vi "TOP LEVEL VI.vi"() -> ()   [LabVIEW 2013]
doc: "This Continuous Measurement sample project is based on the Queued Message Handler template.\n\nThe Event Handling Loop generates messages based on user interface actions.\n\nThe Message Handling Loop processes messages generated by the Event Handling Loop, or by other messages. There are also Acquisition and Logging message handling loop subVIs, and a chart updating loop."
uses:
  Typedefs/Objective selector control enum.ctl
  Typedefs/Laser control knob.ctl
  Typedefs/PMT control knob.ctl
  Typedefs/Frame Size.ctl
  Typedefs/AOL modes.ctl
  Peripherals Control/XYZ Stage/Typedefs/XYZ channel ring.ctl
  Typedefs/Plane Mode.ctl
  Typedefs/AVI implementation enum.ctl
  Typedefs/UI ctrl refs cluster.ctl
  User Interface/Typedefs/Next state queue data.ctl
  Typedefs/Start-Stop Enum.ctl
  Typedefs/Top level VI states.ctl
  Typedefs/Shutter Function Enum.ctl
  <vilib>/Utility/error.llb/DialogType.ctl
  Logging/Globals/gl_Binary timelapse files globals.vi
  Peripherals Control/Pockels/Globals/gl_Pockels control globals.vi
  Global Variables/General Globals.vi
  Global Variables/gl_UI Ctrl Refs.vi
panel:
  in  "Dummy button":bool
  in  "Speed Logging":bool
  in  "Time Lapse":bool
  in  "Live Imaging":bool
  in  "Axis":T1="All" caption="Axis to zero"
  in  "Return to Origin":bool
  out "Stage XYZ Position":cluster{"X":sgl, "Y":sgl, "Z":sgl} caption="Current Stage Position (µm)" {"Z" format="Z:%#_g"; "Y" format="Y:%#_g"; "X" format="X:%#_g"}
  out "Stop":bool=TRUE
  in  "Field of View":sgl(ring)=4.35 items=["175 um"=4.35, "250 um"=5.7, "350 um"=8.7]
  in  "AOL Mode":T2
  in  "Frame Size":T3=512 items=["100X100"=100, "128X128"=128, "200X200"=200, "256X256"=256, "512X512"=512, "1024x1024"=1024, "2048x2048"=2048]
  in  "Objective":T4="Olympus  20X"
  in  "Funct Acq button":bool
  in  "Motor Z Stack":bool
  in  "AOL Z Stack":bool
  in  "Exit button":bool
  in  "Imaging Param Tab":T5(tab)
  out "Power after objective (ind.)":dbl format="%#.0fmW"
  in  "Laser Power":T6=20 caption="LASER" max=1000 step=1 scale=0.0..100.0 scale format="%.0f%"
  out "Back aperture power (ind.)":dbl format="%#.0fmW"
  in  "AOL Z":sgl(slide) min=-178.5 max=177.65 step=0.01 scale=-178.5..177.65 scale format="%#_2f"
  in  "PMT 1":T7=550 max=1000 step=5 scale=0.0..1000.0
  in  "PMT 2":T7=550 max=1000 step=5 scale=0.0..1000.0
  in  "Averages":u16(knob) max=16 step=1 scale=0.0..16.0
  in  "Zoom":i8(slide)=1 min=1 max=24 step=1 scale=1.0..24.0
  in  "Dwell Time":dbl=0.10000000149011612 min=0.05 max=12.0 step=0.05000000074505806 format="%#.2fµs"
  out "Results Directory Overlay":string
  in  "Paths & Names":T8
  in  "Obtain Z Stop":bool
  in  "Obtain Z Start":bool
  in  "# Planes":u16=21 min=1 max=1000
  in  "Pockels@Z Stop":u16=5 caption="Laser % at Z Stop" max=100 format="%.0f%"
  in  "Pockels@Z Start":u16=5 caption="Laser % at Z Start" max=100 format="%.0f%"
  in  "Z Step":dbl=2.0 min=0.1 max=500.0 step=0.1 format="%#.1fµm"
  in  "Z Stop":dbl=-25.0 step=1.0 format="%#.0fµm"
  in  "Z Start":dbl=25.0 step=1.0 format="%#.0fµm"
  out "Center freq ind (nm)":dbl caption="Center frequency" min=800.0 max=1080.0 step=1.0 format="%#.2f MHz"
  in  "Enable f.acq post-processing":bool=TRUE
  in  "Video Record-Funct acq":bool
  in  "Video Record-Live Imaging":bool
  in  "Enable Video Recording":bool
  in  "Virtual Shutter":bool
  in  "Hard Shutter":bool
  in  "Plane Mode":T9 items=["XY Plane"]
  in  "Angle (degrees)":dbl caption="Angle" min=-180.0 max=180.0 format="%#_g°"
  in  "Y centre":dbl min=-1.0 max=1.0 step=0.1 format="%#.2f"
  in  "X centre":dbl min=-1.0 max=1.0 step=0.1 format="%#.2f"
  out "Laser wavelength ind (nm)":dbl caption="Laser wavelength" min=800.0 max=1080.0 step=1.0 format="%#.0f nm"
  in  "Live stim.trig.period":dbl=10.0 caption="Stimulus trigger period" min=0.001 max=50.0 step=1.0 format="%#.6f s"
  in  "Live stim.trig.enable":bool caption="Enable stimulus"
  in  "Funct. Acq. Pockels Modulation":bool caption="Pockels modulation"
  in  "AVI implementation":T10=enum."AVI2"
  in  "Snapshot":bool
  in  "Clear AOL GL":bool
  in  "Abort":bool caption="Stop"
  out "Last State (Ind.)":string
  in  "Switch user":bool
  out "Experiment folder path (ind.)":path caption="Generated experiment folder"
  out "Logging queue (ind)":i32 caption="Elements accumulating\nin the logging queue"
  out "AOL Z-stack Chirps Ready (ind)":bool
  out "Status ind":string
  # "Shutters"
  # "Post-Processing Options"
  # "Cameras Video Recording"
  # "Stimulus Trigger (Live protocols only)"
  # "Debugging Controls (Do not use)"
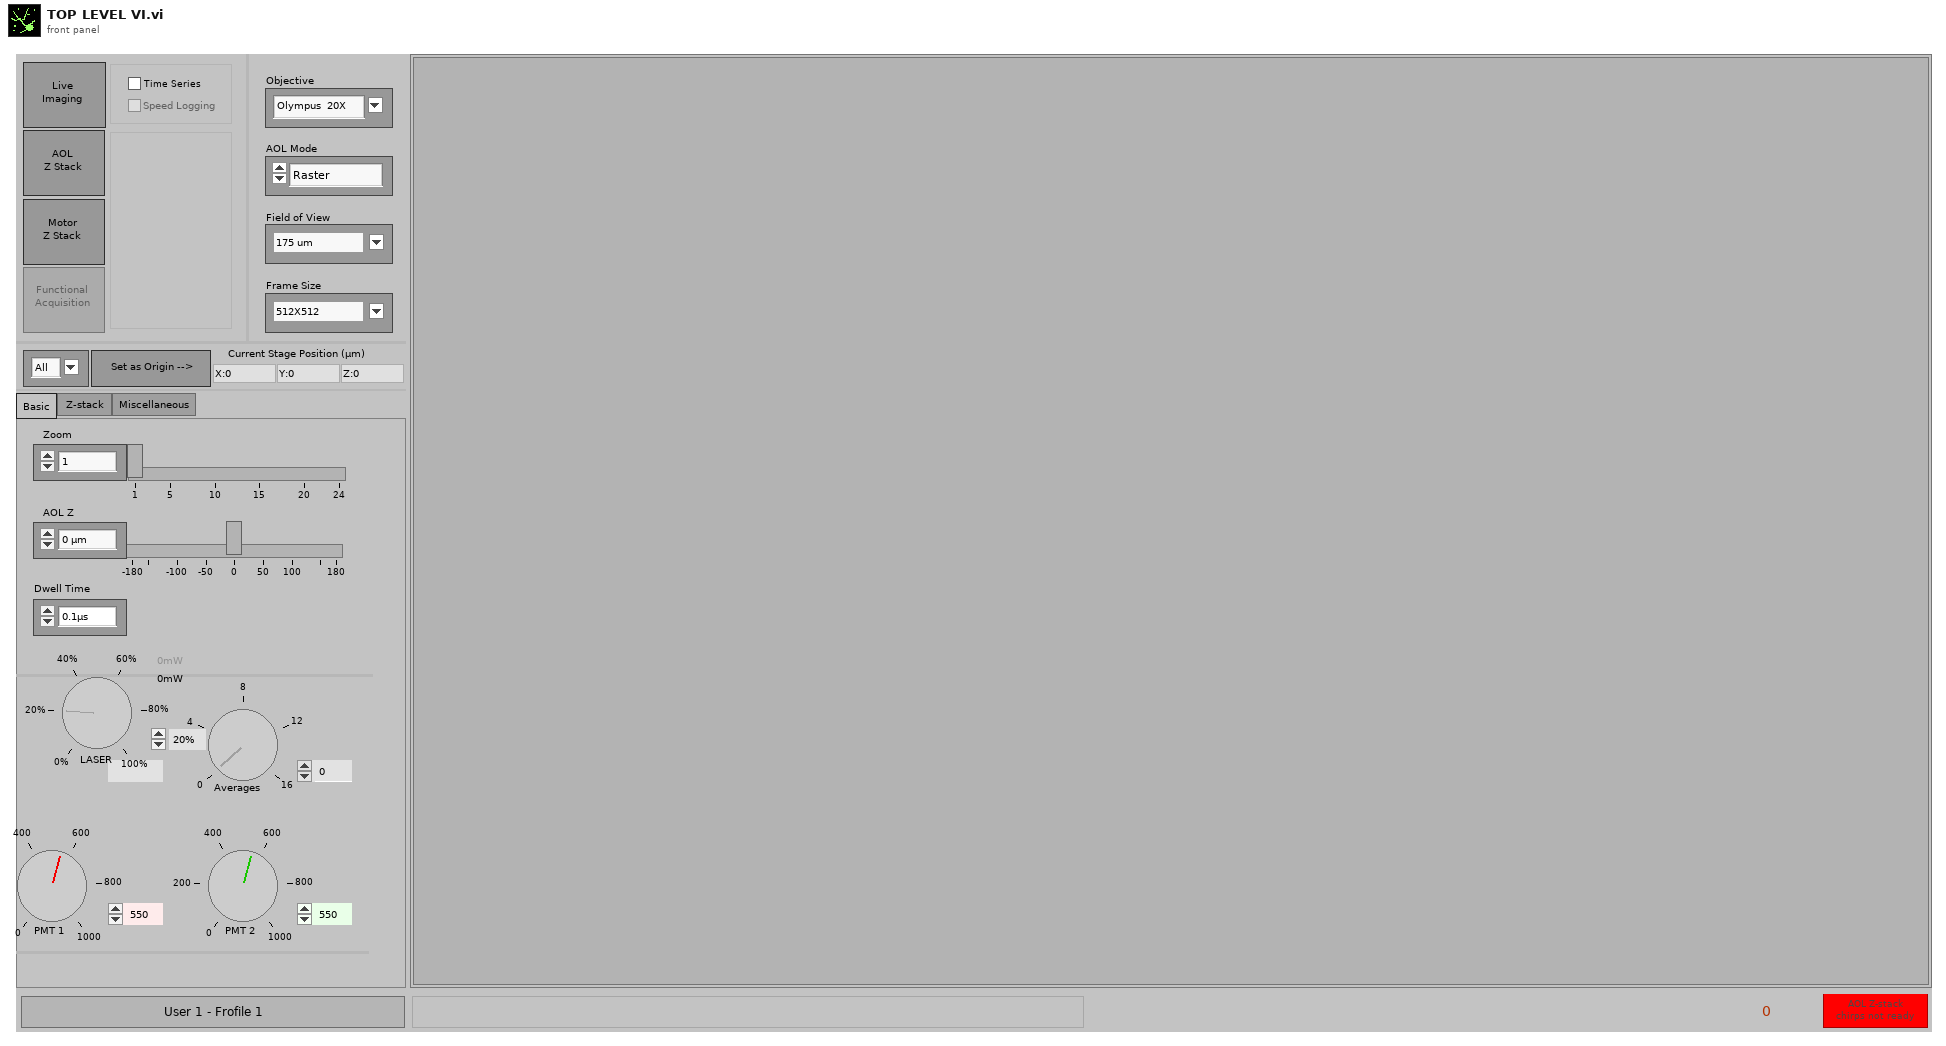
[diagram p1: front panel]
types:
  T1 = typedef "XYZ channel ring.ctl" = string
  T2 = typedef "AOL modes.ctl" = enum16{"Raster", "Structural", "Pointing", "Mini Scan", "Alignment"}
  T3 = typedef "Frame Size.ctl" = u16
  T4 = typedef "Objective selector control enum.ctl" = string
  T5 = enum32{"Basic", "Z-stack ", "Miscellaneous", "Development"}
  T6 = typedef "Laser control knob.ctl" = u16
  T7 = typedef "PMT control knob.ctl" = u16
  T8 = cluster{"Base Directory":path, "User folder?":bool, "Sub-Folder":string, "Experiment folder custom name":string}
  T9 = typedef "Plane Mode.ctl" = u16
  T10 = typedef "AVI implementation enum.ctl" = enum16{"AVI1", "AVI2"}
  T11 = typedef "UI ctrl refs cluster.ctl" = cluster{"Top level VI path":path, "Top level VI ref":refnum<vi>, "User menu ref":refnum<k9>, "Sub Panel control":refnum<vi>, "Imaging Param Tab":refnum<vi>, "Occurrence-Start drivers":refnum<k4>, "Occurrence-Speed logging initialised":refnum<k4>, "Occurrence-XYZ stage initialised":refnum<k4>, "Exit button":refnum<vi>, "Status ind":refnum<vi>, "Return to Origin":refnum<vi>, "Speed Logging":refnum<vi>, "Time Lapse":refnum<vi>, "Live Imaging":refnum<vi>, "AOL Z Stack":refnum<vi>, "Motor Z Stack":refnum<vi>, "Funct Acq button":refnum<vi>, "Hard Shutter":refnum<vi>, "Virtual Shutter":refnum<vi>, "Laser Power":refnum<vi>, "AOL Mode":refnum<vi>, "Frame Size":refnum<vi>, "Field of View":refnum<vi>, "Dwell Time":refnum<vi>, "Zoom":refnum<vi>, "AOL Z":refnum<vi>, "Objective":refnum<vi>, "Axis":refnum<vi>, "Paths & Names":refnum<vi>, "Experiment folder path (ind.)":refnum<vi>, "Last State (Ind.)":refnum<vi>, "Laser wavelength ind (nm)":refnum<vi>, "Averages":refnum<vi>, "Angle (degrees)":refnum<vi>, "X centre":refnum<vi>, "Y centre":refnum<vi>, "Plane Mode":refnum<vi>, "# Planes":refnum<vi>, "Z Start":refnum<vi>, "Z Stop":refnum<vi>, "Z Step":refnum<vi>, "PMT 1":refnum<vi>, "PMT 2":refnum<vi>, "Stage XYZ Position":refnum<vi>, "Pockels@Z Start":refnum<vi>, "Pockels@Z Stop":refnum<vi>, "Obtain Z Start":refnum<vi>, "Obtain Z Stop":refnum<vi>, "Live stim.trig.period":refnum<vi>, "Live stim.trig.enable":refnum<vi>, "Funct. Acq. Pockels Modulation":refnum<vi>, "Enable Video Recording":refnum<vi>, "Video Record-Live Imaging":refnum<vi>, "Video Record-Funct acq":refnum<vi>, "AOL Z-stack Chirps Ready (ind)":refnum<vi>, "Center freq ind (nm)":refnum<vi>, "Logging queue (ind)":refnum<vi>, "Back aperture power (ind.)":refnum<vi>, "Power after objective (ind.)":refnum<vi>, "Switch user":refnum<vi>}
  T12 = enum8{"Enabled", "Disabled", "Disabled and Grayed Out"}
  T13 = typedef "Next state queue data.ctl" = cluster{"Start/Stop":T14, "State":T15}
  T14 = typedef "Start-Stop Enum.ctl" = enum16{"START", "STOP"}
  T15 = typedef "Top level VI states.ctl" = enum16{"None", "Initialise UI", "<STACK PROTOCOL STATES>", "AOL Zstack-START", "AOL Zstack-STOP", "Motor Zstack-START", "Motor Zstack-STOP", "<ACQUISITION PROTOCOL STATES> ", "Functional Acquisition-START", "Functional Acquisition-STOP", "Single Plane Acquisition-START", "Single Plane Acquisition-STOP", "Volume Acquisition-START", "Volume Acquisition-STOP", "<LIVE IMAGING PROTOCOL STATES>", "Live Imaging-START", "Live Imaging-STOP", "Live Plane Imaging-START", "Live Plane Imaging-STOP", "Live Volume Imaging-START", "Live Volume Imaging-STOP", "EXIT"}
  T16 = enum16{"Write Red AVI", "Write Green AVI", "Write AVI mode"}
  T17 = typedef "Shutter Function Enum.ctl" = enum16{"Open Shutter", "Close Shutter"}
  T18 = enum16{"Software Init", "User menu", "Switch User button"}
  T19 = typedef "All Message Queues.ctl" = cluster{"UI queue":refnum<queue>, "Acq. queue":refnum<queue>, "Logging queue":refnum<queue>}
  T20 = typedef "DialogType.ctl" = u16
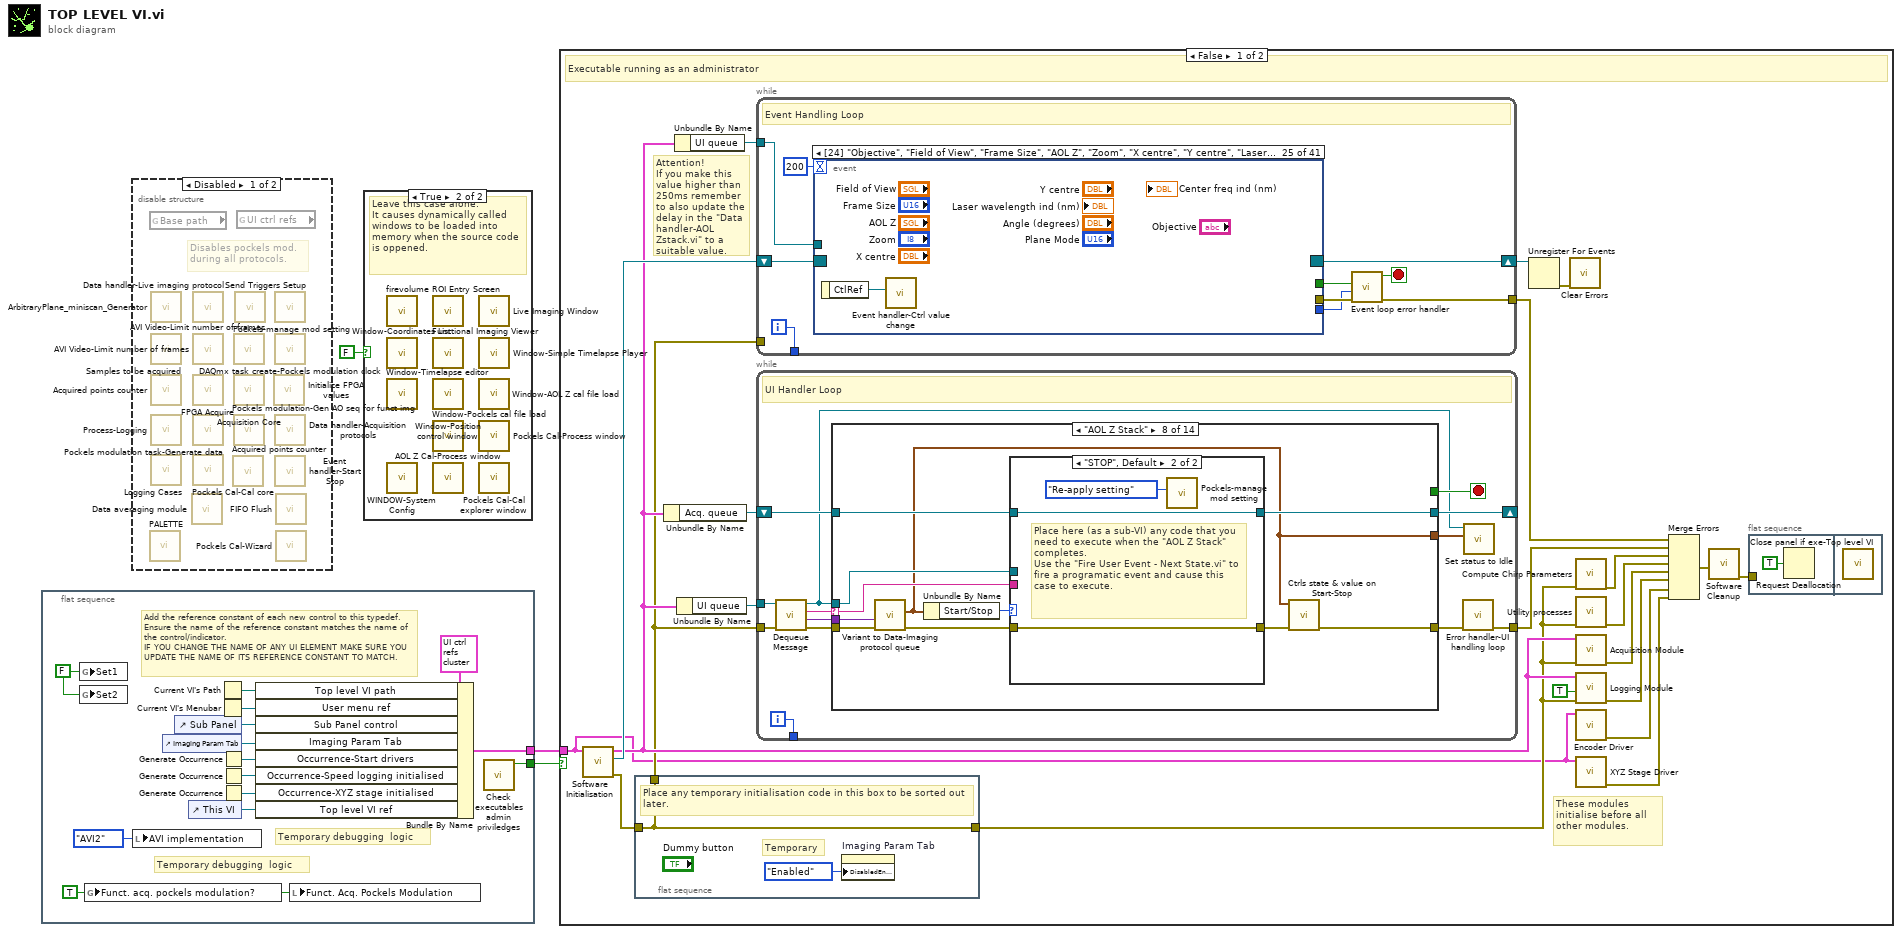
[diagram p0: block diagram]
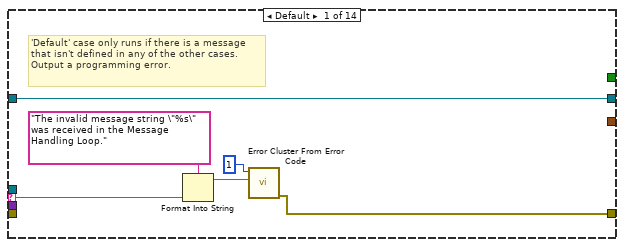
[diagram p2: hidden frame]
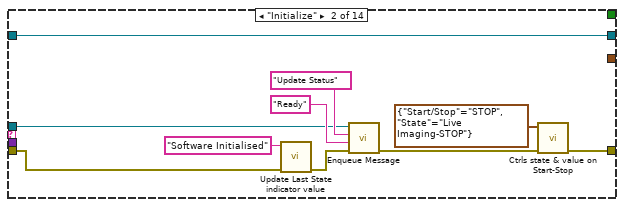
[diagram p3: hidden frame]
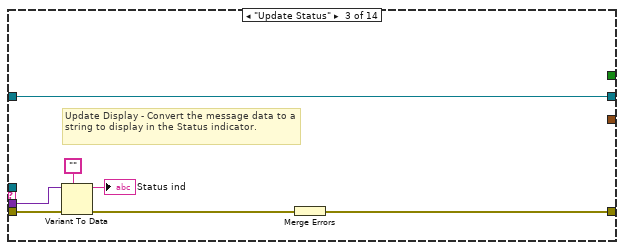
[diagram p4: hidden frame]
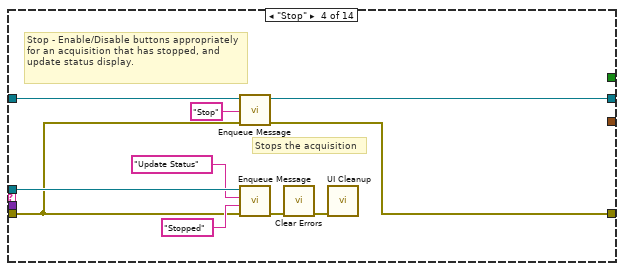
[diagram p5: hidden frame]
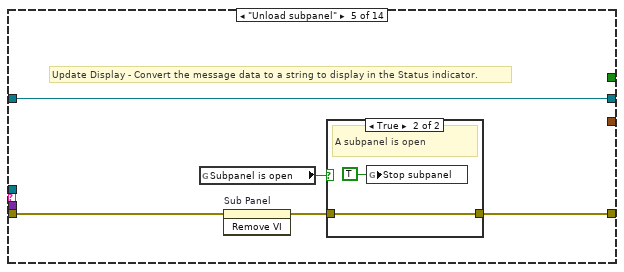
[diagram p6: hidden frame]
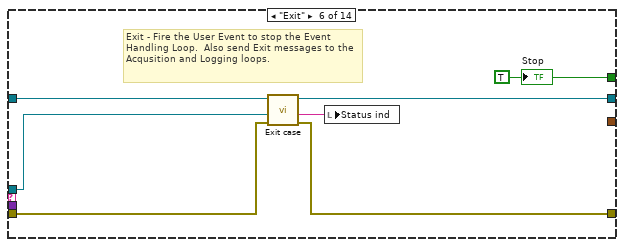
[diagram p8: hidden frame]
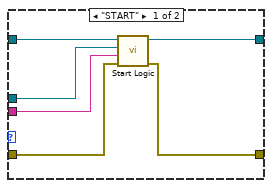
[diagram p10: hidden frame]
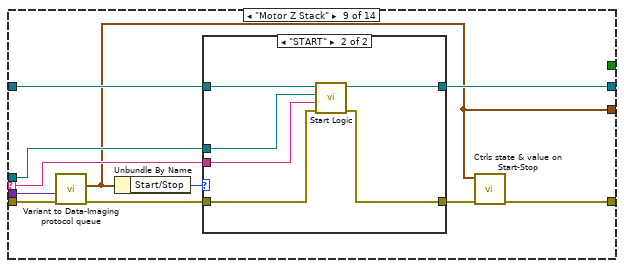
[diagram p11: hidden frame]
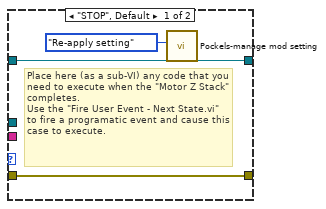
[diagram p12: hidden frame]
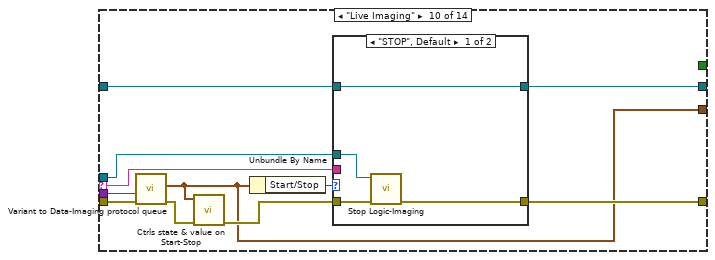
[diagram p13: hidden frame]
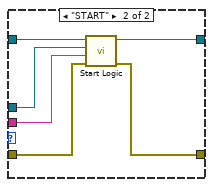
[diagram p14: hidden frame]
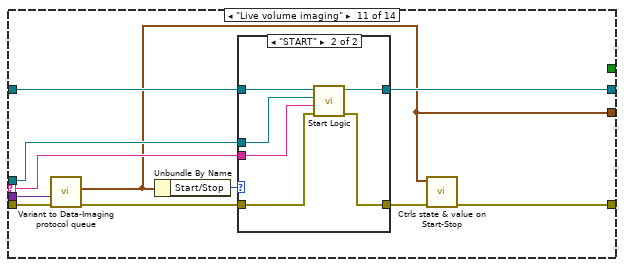
[diagram p15: hidden frame]
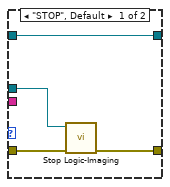
[diagram p16: hidden frame]
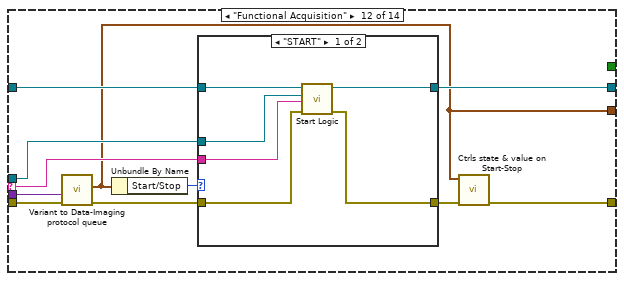
[diagram p17: hidden frame]
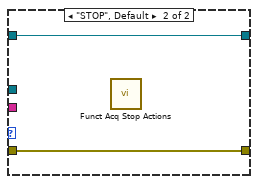
[diagram p18: hidden frame]
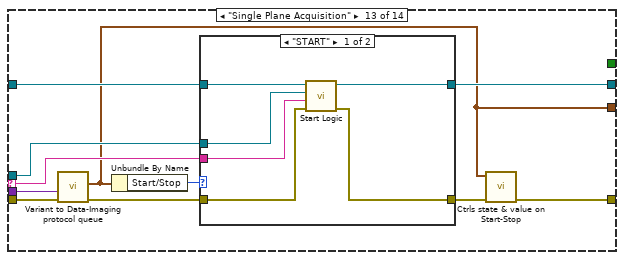
[diagram p19: hidden frame]
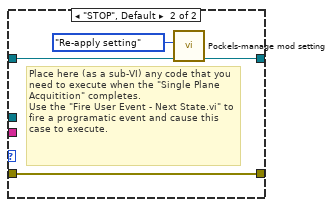
[diagram p20: hidden frame]
diagram:
  n1 = flat-sequence {
    tunnel: [w17] -> w2
    tunnel: [w4] -> w1
    frame #0 {
      w7 = TRUE ("Funct. acq. pockels modulation?")
      w9 = FALSE ("Set1")
      # "Temporary debugging  logic"
      # "Temporary debugging  logic"
      # "Add the reference constant of each new control to this typedef. Ensure the name of the reference constant matches the name of the control/indicator.\nIF YOU CHANGE THE NAME OF ANY UI ELEMENT MAKE SURE YOU UPDATE THE NAME OF ITS REFERENCE CONSTANT TO MATCH."
      n2 = global write "gl_Binary timelapse files globals.vi" "Set1"(w9) -> ()
      n3 = global write "gl_Binary timelapse files globals.vi" "Set2"(w9) -> ()
      n4 = global write "gl_Pockels control globals.vi" "Funct. acq. pockels modulation?"(w7) -> ()
      n5 = local write "AVI implementation"(AVI_implementation_enum."AVI2" ("AVI implementation")) -> ()
      n6 = control-ref of="Imaging Param Tab"() -> (w13:refnum<vi>)
      n7 = control-ref of="Sub Panel"() -> (w5:refnum<vi>)
      n8 = control-ref of="This VI"() -> (w10:refnum<vi>)
      n9 = Current VI's Path() -> (path=w15:path)
      n10 = Current VI's Menubar() -> (w16:refnum<k9>)
      n11 = Generate Occurrence() -> (w6:refnum<k4>)
      n12 = Generate Occurrence() -> (w11:refnum<k4>)
      n13 = Generate Occurrence() -> (w12:refnum<k4>)
      n14 = Bundle By Name(cluster=T11 {"Top level VI path"=path "", "Top level VI ref"=refnum, "User menu ref"=refnum, "Sub Panel control"=refnum, "Imaging Param Tab"=refnum, "Occurrence-Start drivers"=refnum, "Occurrence-Speed logging initialised"=refnum, "Occurrence-XYZ stage initialised"=refnum, "Exit button"=refnum, "Status ind"=refnum, "Return to Origin"=refnum, "Speed Logging"=refnum, "Time Lapse"=refnum, "Live Imaging"=refnum, "AOL Z Stack"=refnum, "Motor Z Stack"=refnum, "Funct Acq button"=refnum, "Hard Shutter"=refnum, "Virtual Shutter"=refnum, "Laser Power"=refnum, "AOL Mode"=refnum, "Frame Size"=refnum, "Field of View"=refnum, "Dwell Time"=refnum, "Zoom"=refnum, "AOL Z"=refnum, "Objective"=refnum, "Axis"=refnum, "Paths & Names"=refnum, "Experiment folder path (ind.)"=refnum, "Last State (Ind.)"=refnum, "Laser wavelength ind (nm)"=refnum, "Averages"=refnum, "Angle (degrees)"=refnum, "X centre"=refnum, "Y centre"=refnum, "Plane Mode"=refnum, "# Planes"=refnum, "Z Start"=refnum, "Z Stop"=refnum, "Z Step"=refnum, "PMT 1"=refnum, "PMT 2"=refnum, "Stage XYZ Position"=refnum, "Pockels@Z Start"=refnum, "Pockels@Z Stop"=refnum, "Obtain Z Start"=refnum, "Obtain Z Stop"=refnum, "Live stim.trig.period"=refnum, "Live stim.trig.enable"=refnum, "Funct. Acq. Pockels Modulation"=refnum, "Enable Video Recording"=refnum, "Video Record-Live Imaging"=refnum, "Video Record-Funct acq"=refnum, "AOL Z-stack Chirps Ready (ind)"=refnum, "Center freq ind (nm)"=refnum, "Logging queue (ind)"=refnum, "Back aperture power (ind.)"=refnum, "Power after objective (ind.)"=refnum, "Switch user"=refnum} ("output cluster"), "Top level VI path"=w15, "User menu ref"=w16, "Sub Panel control"=w5, "Imaging Param Tab"=w13, "Occurrence-Start drivers"=w6, "Occurrence-Speed logging initialised"=w11, "Occurrence-XYZ stage initialised"=w12, "Top level VI ref"=w10) -> (w17:T11)
      n15 = local write "Funct. Acq. Pockels Modulation"(w7) -> ()
      n16 = call "Check executables admin priviledges.vi"() -> ("Exe not run as an administrator"=w4:bool)  [unwired: 10 in, 1 out]
    }
  }
  n17 = disable-structure shown="Disabled" {
    frame Disabled {
      # "Disables pockels mod.\nduring all protocols."
      n18 = global read "General Globals.vi" "Base path"() -> ()  [unwired: 1 out]
      n19 = call "PALETTE.vi"() -> ()  [unwired: 12 in]
      n20 = call "ArbitraryPlane_miniscan_Generator.vi"() -> ()  [unwired: 7 in, 5 out]
      n21 = call "Samples to be acquired.vi"() -> ()  [unwired: 10 in, 2 out]
      n22 = call "Acquired points counter.vi"() -> ()  [unwired: 12 in, 4 out]
      n23 = call "Process-Logging.vi"() -> ()  [unwired: 11 in, 1 out]
      n24 = call "Logging Cases.vi"() -> ()  [unwired: 14 in, 2 out]
      n25 = call "Data averaging module.vi"() -> ()  [unwired: 8 in, 4 out]
      n26 = call "Data handler-Live imaging protocol.vi"() -> ()  [unwired: 15 in, 1 out]
      n27 = call "AVI Video-Limit number of frames.vi"() -> ()  [unwired: 1 in, 1 out]
      n28 = call "FPGA Acquire.vi"() -> ()  [unwired: 11 in, 5 out]
      n29 = call "Pockels modulation task-Generate data.vi"() -> ()  [unwired: 7 in, 5 out]
      n30 = call "Pockels Cal-Cal core.vi"() -> ()  [unwired: 9 in, 3 out]
      n31 = call "Acquired points counter.vi"() -> ()  [unwired: 12 in, 4 out]
      n32 = call "AVI Video-Limit number of frames.vi"() -> ()  [unwired: 1 in, 1 out]
      n33 = call "Acquisition Core.vi"() -> ()  [unwired: 10 in, 2 out]
      n34 = call "Pockels modulation-Gen AO seq for funct img.vi"() -> ()  [unwired: 8 in, 4 out]
      n35 = call "Pockels-manage mod setting.vi"() -> ()  [unwired: 11 in, 1 out]
      n36 = global read "gl_UI Ctrl Refs.vi" "UI ctrl refs"() -> ()  [unwired: 1 out]
      n37 = call "Initialize FPGA values.vi"() -> ()  [unwired: 10 in, 2 out]
      n38 = call "Send Triggers Setup.vi"() -> ()  [unwired: 10 in, 2 out]
      n39 = call "DAQmx task create-Pockels modulation clock.vi"() -> ()  [unwired: 10 in, 2 out]
      n40 = call "Data handler-Acquisition protocols.vi"() -> ()  [unwired: 14 in, 2 out]
      n41 = call "Event handler-Start Stop.vi"() -> ()  [unwired: 10 in, 2 out]
      n42 = call "FIFO Flush.vi"() -> ()  [unwired: 9 in, 3 out]
      n43 = call "Pockels Cal-Wizard.vi"() -> ()  [unwired: 12 in]
    }
    frame Enabled {
    }
  }
  n44 = case shown="True" FALSE {
    frame False {
    }
    frame True {
      # "Leave this case alone.\nIt causes dynamically called windows to be loaded into memory when the source code is oppened."
      n45 = call "firevolume.vi"() -> ()  [unwired: 12 in]
      n46 = call "Window-Coordinates List.vi"() -> ()  [unwired: 12 in]
      n47 = call "Window-Timelapse editor.vi"() -> ()  [unwired: 12 in]
      n48 = call "WINDOW-System Config.vi"() -> ()  [unwired: 12 in]
      n49 = call "ROI Entry Screen.vi"() -> ()  [unwired: 12 in]
      n50 = call "Functional Imaging Viewer.vi"() -> ()  [unwired: 12 in]
      n51 = call "Window-Position control window.vi"() -> ()  [unwired: 12 in]
      n52 = call "Window-Pockels cal file load.vi"() -> ()  [unwired: 12 in]
      n53 = call "AOL Z Cal-Process window.vi"() -> ()  [unwired: 9 in, 3 out]
      n54 = call "Live Imaging Window.vi"() -> ()  [unwired: 12 in]
      n55 = call "Window-Simple Timelapse Player.vi"() -> ()  [unwired: 12 in]
      n56 = call "Window-AOL Z cal file load.vi"() -> ()  [unwired: 12 in]
      n57 = call "Pockels Cal-Process window.vi"() -> ()  [unwired: 10 in, 2 out]
      n58 = call "Pockels Cal-Cal explorer window.vi"() -> ()  [unwired: 12 in]
    }
  }
  n59 = case shown="False" w1 {
    tunnel: w2 -> [w18 w319]
    frame False {
      # "These modules initialise before all other modules."
      # "Attention!\nIf you make this value higher than 250ms remember to also update the delay in the \"Data handler-AOL Zstack.vi\" to a suitable value."
      # "Executable running as an administrator"
      n60 = call "Software Initialisation.vi"("UI elements cluster"=w18) -> ("Error Out"=w37:errorcluster, "Event Registration Refnum"=w39:refnum<event-registration>, "Message Queues out"=w38:T19)  [unwired: 8 in]
      n61 = flat-sequence {
        tunnel: w37 -> [w41]
        tunnel: [w41] -> w21
        tunnel: [w41] -> w20
        frame #0 {
          # "Temporary"
          # "Place any temporary initialisation code in this box to be sorted out later."
          n62 = property on="Imaging Param Tab" class="TabCtl (strict)"("DisabledEnum"=T12."Enabled" ("Disabled")) -> ()  [unwired: 2 in, 2 out]
        }
      }
      n63 = Unbundle By Name(w38) -> ("Acq. queue"=w33:refnum<queue>)
      n64 = Unbundle By Name(w38) -> ("UI queue"=w35:refnum<queue>)
      n65 = Unbundle By Name(w38) -> ("UI queue"=w34:refnum<queue>)
      n66 = while {
        tunnel: w35 -> [w253]
        tunnel: [w251] -> w26
        shift-right: [w252] -> w36
        shift-left: w39 -> [w254]
        tunnel: [w248] -> _
        tunnel: w21 -> [_]
        i -> [w248]
        stop <- w256 stop-if-true
        # "Event Handling Loop"
        n67 = event shown="[24] \"Objective\", \"Field of View\", \"Frame Size\", \"AOL Z\", \"Zoom\", \"X centre\", \"Y centre\", \"Laser wavelength ind (nm)\", \"Angle (degrees)\", \"Plane Mode\": Value Change" {
          selector: w254 -> [_ _ _ _ _ _ _ _ _ _ _ _ _ _ _ _ _ _ _ _ _ _ _ _ _ _ _ _ _ _ _ _ _ _ _ _ _ _ _ _ _]
          dyn-events: [_ _ _ _ _ _ _ _ _ _ _ _ _ _ _ _ _ _ _ _ _ _ _ _ _ _ _ _ _ _ _ _ _ _ _ _ _ _ _ _ _] -> w252
          timeout: 200 -> [_ _ _ _ _ _ _ _ _ _ _ _ _ _ _ _ _ _ _ _ _ _ _ _ _ _ _ _ _ _ _ _ _ _ _ _ _ _ _ _ _]
          tunnel: [_ _ _ _ _ _ _ _ _ _ _ _ _ _ _ _ _ _ _ _ _ _ _ _ _ _ _ _ _ _ _ _ _ _ _ _ _ _ TRUE ("Discard?") _ _] -> w249
          tunnel: w253 -> [_ w258 _ _ w263 _ _ _ _ _ _ _ _ _ _ _ _ _ _ _ _ _ _ _ _ _ _ _ _ _ _ _ _ _ _ _ _ w311 _ w314 w317]
          tunnel: [_ w257 _ _ w262 _ _ _ w268 w273 w275 w277 _ _ w281 _ _ _ _ _ _ _ _ _ _ _ _ _ _ _ _ _ _ _ _ _ _ w310 _ w315 w318] -> w255
          tunnel: [_ _ _ _ w261 _ _ _ _ _ _ _ _ _ _ _ _ _ _ _ _ _ _ _ _ _ _ _ _ _ _ _ _ _ _ _ _ _ _ _ _] -> w247
          event Timeout {
            n68 = event-data() -> ()  [unwired: 1 in, 1 out]
          }
          event Menu Selection (User); "Experiment folder path (ind.)", "Results Directory Overlay": Shortcut Menu Selection (User) {
            n69 = event-data() -> ("ItemTag"=w259:string)  [unwired: 1 in]
            n70 = call "User menu handler.vi"("UI queue"=w258, "User Menu ItemTag"=w259) -> ("error out"=w257:errorcluster)  [unwired: 9 in]
          }
          event "Live stim.trig.period", "Return to Origin", "Laser wavelength ind (nm)": Shortcut Menu Selection (User) {
            n71 = event-data() -> ("ItemTag"=w260:string)  [unwired: 1 in]
            n72 = call "Top level UI-Shortcut menus handler.vi"("ItemTag"=w260) -> ()  [unwired: 11 in]
          }
          event Menu Activation? {
            n73 = event-data() -> ()  [unwired: 1 in, 5 out]
            n74 = call "menu-Cal group disabled state.vi"() -> ()  [unwired: 10 in, 2 out]
            n75 = event-data() -> ()  [unwired: 2 in, 1 out]
          }
          event User Event {
            # "Causes the \"UI Handler Loop\" to execute one of its cases. There are redundant cases as a provision.\nThis functionality is fully scalable and flexible allowing to programatically fire events from anywhere within the software, as well as when the user presses a button.\nThis event case also executes in response to a programmatic event which occurs when the user closes the ROI Entry Screen, and executes the required case, depending on which button the user pressed to exit the ROI Entry Screen."
            n76 = event-data() -> ("Next State"=w261:T15)  [unwired: 1 in]
            n77 = call "Event handler-Start Stop.vi"("Next State"=w261, "UI queue"=w263) -> ("error out"=w262:errorcluster)  [unwired: 8 in, 1 out]
          }
          event "Experiment folder path (ind.)": Shortcut Menu Activation? {
            n78 = event-data() -> ("CtlRef"=w266:refnum<vi>)  [unwired: 1 in]
            n79 = property class="Path"(reference=w266) -> ("Value"=w265:path)  [unwired: 1 in, 2 out]
            n80 = Empty String/Path?(string/path=w265) -> (empty?=w264:bool)
            n81 = event-data("Discard?"=w264) -> ()  [unwired: 1 in, 1 out]
          }
          event "Live stim.trig.enable", "Live stim.trig.period": Value Change {
            n82 = event-data() -> ()  [unwired: 1 in, 1 out]
            n83 = call "Stimulus trigger period event handler.vi"() -> ()  [unwired: 12 in]
          }
          event "Enable f.acq post-processing": Value Change {
            n84 = event-data() -> ("NewVal"=w267:bool)  [unwired: 1 in]
            n85 = global write "General Globals.vi" "Funct.acq post-proc enabled"(w267) -> ()
          }
          event "Live Imaging": Value Change {
            # "Sends the \" <Next state>:User Event \" case of this event structure to its specified sub-case."
            n86 = event-data() -> ("NewVal"=w272:bool)  [unwired: 1 in]
            n87 = Select(t=Top_level_VI_states."Live Imaging-START" ("event data / imaging mode"), s=w272, f=Top_level_VI_states."Live Imaging-STOP" ("event data / imaging mode")) -> (s? t:f=w270:T15)
            n88 = call "Fire User Event - Next State.vi"("\"UI Handler loop\" case to execute"=w270) -> ("Error Out"=w268:errorcluster)  [unwired: 10 in]
          }
          event "AOL Z Stack": Value Change {
            n89 = event-data() -> ("NewVal"=w274:bool)  [unwired: 1 in]
            n90 = call "Event handler-AOL Z button.vi"("AOL Z button's value"=w274) -> ("error out"=w273:errorcluster)  [unwired: 10 in]
          }
          event "Motor Z Stack": Value Change {
            n91 = event-data() -> ("NewVal"=w276:bool)  [unwired: 1 in]
            n92 = call "Event handler-Motor Z button.vi"("Motor Z button's value"=w276) -> ("error out"=w275:errorcluster)  [unwired: 10 in]
          }
          event "Funct Acq button": Value Change {
            n93 = event-data() -> ("NewVal"=w278:bool)  [unwired: 1 in]
            n94 = call "Event handler-Funct Acq button.vi"("Funct.Acq button's value"=w278) -> ("error out"=w277:errorcluster)  [unwired: 10 in]
          }
          event "Paths & Names.Base Directory": Value Change {
            n95 = event-data() -> ("OldVal"=w279:path)  [unwired: 1 in]
            n96 = call "Event handler-Dir change.vi"("Old Base Path"=w279) -> ()  [unwired: 11 in]
          }
          event "Paths & Names.User folder?": Value Change {
            n97 = event-data() -> ("NewVal"=w280:bool)  [unwired: 1 in]
            n98 = global write "General Globals.vi" "Generate user folder?"(w280) -> ()
          }
          event "Time Lapse": Value Change {
            n99 = event-data() -> ()  [unwired: 1 in, 1 out]
            n100 = call "Event handler-Timelapse.vi"() -> ("error out"=w281:errorcluster)  [unwired: 11 in]
          }
          event "Enable Video Recording": Value Change {
            n101 = event-data() -> ("NewVal"=w282:bool)  [unwired: 1 in]
            n102 = call "Event handler-VidRec enable.vi"("Enable Video Recording.NewVal"=w282) -> ()  [unwired: 11 in]
          }
          event "Video Record-Live Imaging": Value Change {
            n103 = event-data() -> ("NewVal"=w283:bool)  [unwired: 1 in]
            n104 = call "Event handler-VidRec enable in timelapse.vi"("Video Record-Live Imaging.NewVal"=w283) -> ()  [unwired: 11 in]
          }
          event "Video Record-Funct acq": Value Change {
            n105 = event-data() -> ("NewVal"=w284:bool)  [unwired: 1 in]
            n106 = call "Event handler-VidRec enable in funct.vi"("Video Record-Funct acq.NewVal"=w284) -> ()  [unwired: 11 in]
          }
          event Value Change {
            n107 = event-data() -> ("NewVal"=w285:T10)  [unwired: 1 in]
            n108 = call "fgv_AVI_Globals.vi"("AVI mode"=w285, "Function"=enum16{"Intialize", "Write", "Read", "Clear"}."Write", "\"Write\" sub function"=T16."Write AVI mode" ("\"Write\" sub function")) -> ()  [unwired: 9 in, 4 out]
          }
          event "Snapshot": Value Change {
            # "Warning! Redundant case. Eliminate if no longer needed."
            n109 = event-data() -> ()  [unwired: 1 in, 1 out]
            n110 = disable-structure shown="Disabled" {
              frame Disabled {
                # "Right graph data"
                # "Left graph data"
                # "As soon as this button is pressed this code grabs both the left and right graph data (each being a 2D array of points) and saves it to the file specified by the user in a pop up file-dialogue window."
                n111 = call "Intensity Graphs to Excel.vi"() -> ()  [unwired: 12 in]
              }
              frame Enabled {
              }
            }
          }
          event "Obtain Z Start", "Obtain Z Stop", "Z Step", "Z Start", "Z Stop": Value Change {
            n112 = event-data() -> ()  [unwired: 1 in, 1 out]
            n113 = call "Event handler-Z Setup.vi"("Obtain Z Stop"="Obtain Z Stop", "Obtain Z Start"="Obtain Z Start") -> ()  [unwired: 9 in, 1 out]
          }
          event "Pockels@Z Start", "Pockels@Z Stop": Value Change {
            n114 = event-data() -> ()  [unwired: 1 in, 1 out]
            n115 = call "Event handler-Z Setup pockels entry.vi"() -> ()  [unwired: 11 in, 1 out]
          }
          event "# Planes": Value Change {
            n116 = event-data() -> ()  [unwired: 1 in, 1 out]
            n117 = call "Event handler-Number of planes change.vi"() -> ()  [unwired: 11 in, 1 out]
          }
          event "Averages": Value Change {
            n118 = event-data() -> ("NewVal"=w290:u16)  [unwired: 1 in]
            n119 = call "Event handler-Averages ValChange.vi"("Averages.NewVal"=w290) -> ()  [unwired: 11 in]
          }
          event "Field of View", "AOL Z", "Zoom", "X centre", "Y centre", "Laser wavelength ind (nm)", "Angle (degrees)": Value Change {
            n120 = event-data() -> ("CtlRef"=w291:refnum<vi>)  [unwired: 1 in]
            n121 = call "Event handler-Ctrl value change.vi"("Control in"=w291) -> ()  [unwired: 11 in]
          }
          event "Dwell Time": Value Change {
            n122 = event-data() -> ()  [unwired: 1 in, 1 out]
            n123 = call "AOL Globals Dwell Time updater.vi"() -> ()  [unwired: 11 in, 1 out]
          }
          event Value Change {
            n124 = event-data() -> ()  [unwired: 1 in, 1 out]
            n125 = call "AOL Globals mode updater.vi"() -> ("error out"=w292:errorcluster)  [unwired: 11 in]
            n126 = call "AOL Globals Dwell Time updater.vi"("error in"=w292) -> ()  [unwired: 10 in, 1 out]
          }
          event "Return to Origin": Value Change {
            n127 = event-data() -> ()  [unwired: 1 in, 1 out]
            n128 = call "Event handler-Set coordinates to zero.vi"() -> ()  [unwired: 12 in]
          }
          event "Hard Shutter": Value Change {
            n129 = event-data() -> ()  [unwired: 1 in, 1 out]
            n130 = Select(t=Shutter_Function_Enum."Open Shutter" ("Shutter Function"), s="Hard Shutter", f=Shutter_Function_Enum."Close Shutter" ("Shutter Function")) -> (s? t:f=w294:T17)
            n131 = call "Set Hard Shutter.vi"("Shutter Function"=w294) -> ("Error Out"=w293:errorcluster)  [unwired: 10 in]
            n132 = case shown="Error" w293 {
              selector: w293 -> [_ w299]
              frame No Error {
              }
              frame Error {
                w300 = T20 0 items=["no dialog", "OK message", "continue or stop message", "OK message + warnings", "continue/stop + warnings"] ("type of dialog (OK msg:1)")
                n133 = call <vilib>:"Simple Error Handler.vi"("type of dialog (OK msg:1)"=w300, "error in (no error)"=w299) -> ("error out"=w298:errorcluster)  [unwired: 3 in, 4 out]
                n134 = call "Window-Error message.vi"("error in (no error)"=w298, "Message"="Hard shutter error") -> ()  [unwired: 9 in, 1 out]
              }
            }
          }
          event Value Change {
            n135 = event-data() -> ("NewVal"=w302:T6)  [unwired: 1 in]
            n136 = call "Event handler-Laser power value change.vi"("Laser Power knob.NewVal"=w302) -> ()  [unwired: 11 in]
          }
          event Mouse Up; Mouse Leave {
            n137 = event-data() -> ()  [unwired: 1 in, 1 out]
            n138 = local read "Laser Power"() -> (w304:T6)
            n139 = To Unsigned Byte Integer(number=w304) -> (unsigned 8bit integer=w303:u8)
            n140 = call "Set laser power.vi"("Laser power %"=w303) -> ()  [unwired: 10 in, 1 out]
          }
          event "Funct. Acq. Pockels Modulation": Value Change {
            n141 = event-data() -> ()  [unwired: 1 in, 1 out]
            n142 = global write "gl_Pockels control globals.vi" "Funct. acq. pockels modulation?"("Funct. Acq. Pockels Modulation") -> ()
          }
          event "Virtual Shutter": Value Change {
            n143 = event-data() -> ("NewVal"=w306:bool)  [unwired: 1 in]
            n144 = call "Event handler-Virtual shutter change.vi"("Virtual shutter button value"=w306) -> ()  [unwired: 11 in]
          }
          event Value Change {
            n145 = event-data() -> ()  [unwired: 1 in, 1 out]
            n146 = call "Event handler-PMT value change.vi"() -> ()  [unwired: 12 in]
          }
          event "Speed Logging": Value Change {
            n147 = event-data() -> ("NewVal"=w307:bool)  [unwired: 1 in]
            n148 = global write "General Globals.vi" "Speed logging enabled"(w307) -> ()
          }
          event "Clear AOL GL": Value Change {
            # "This functionality is only needed during development and it will be eventually eliminated."
            n149 = event-data() -> ()  [unwired: 1 in, 1 out]
            n150 = call "fgv_AOL_Globals.vi"("Function"=enum16{"Intialize", "Write", "Read", "Clear"}."Clear") -> ()  [unwired: 9 in, 2 out]
          }
          event "Switch user": Value Change {
            n151 = event-data() -> ()  [unwired: 1 in, 2 out]
            n152 = call "UsrProfiles-User login.vi"("Access source (Soft init)"=T18."Switch User button") -> ()  [unwired: 10 in, 1 out]
          }
          event "Abort": Value Change {
            n153 = event-data() -> ()  [unwired: 1 in, 1 out]
            n154 = call "Enqueue Message.vi"("Message"="Stop", "Queue"=w311) -> ("error out"=w310:errorcluster)  [unwired: 8 in, 1 out]
          }
          event User Event {
            # "Do not add any code in this case.\nThis case is only used to cause the event loop to stop.\nuse the subVI in the disaboled case below to fire a programmatic event from anywhere, which will stop the event handling loop."
            n155 = event-data() -> ()  [unwired: 1 in, 1 out]
            n156 = disable-structure shown="Enabled" {
              frame Disabled {
                n157 = call "Fire User Event - Stop.vi"() -> ()  [unwired: 11 in, 1 out]
              }
              frame Enabled {
              }
            }
          }
          event "Exit button": Value Change {
            # "The UI Message Loop handles sending the Exit message to other loops."
            n158 = event-data() -> ()  [unwired: 1 in, 1 out]
            n159 = call "Event handler-Exit.vi"("UI queue"=w314) -> ("error out"=w315:errorcluster)  [unwired: 9 in, 1 out]
          }
          event Panel Close? {
            n160 = event-data() -> ()  [unwired: 1 in, 1 out]
            n161 = call "Event handler-Exit.vi"("UI queue"=w317) -> ("error out"=w318:errorcluster)  [unwired: 9 in, 1 out]
            n162 = event-data("Discard?"=TRUE) -> ()  [unwired: 1 in, 1 out]
          }
        }
        n163 = call "Event loop error handler.vi"("error in (no error)"=w255, "Next State"=w247, "Stop?"=w249) -> ("error out"=w251:errorcluster, "Stop event handling loop"=w256:bool)  [unwired: 7 in]
      }
      n164 = while {
        tunnel: w34 -> [w51]
        tunnel: w21 -> [w48]
        tunnel: [w47] -> w22
        shift-right: [w45] -> _
        shift-left: w33 -> [w50]
        tunnel: [w46] -> _
        i -> [w46]
        stop <- w55 stop-if-true
        # "UI Handler Loop"
        n165 = call "Dequeue Message.vi"("Error In"=w48, "Message Queue"=w51) -> ("Error Out"=w54:errorcluster, "Message Data"=w52:variant, "Message"=w53:string, "dup Message Queue"=w43:refnum<queue>)  [unwired: 5 in, 1 out]
        n166 = case "Message Cases" shown="\"AOL Z Stack\"" w53 {
          selector: w53 -> [w60 _ _ _ _ _ _ w107 w127 w153 w169 w189 w209 w228]
          tunnel: w43 -> [_ w66 _ w88 _ w97 _ w116 w136 w149 w177 w194 w217 w233]
          tunnel: w54 -> [_ w69 w77 w83 w90 w103 w105 w115 w135 w156 w176 w196 w216 w235]
          tunnel: [w58 w62 w78 w82 w93 w101 w105 w111 w131 w150 w173 w192 w214 w237] -> w49
          tunnel: [_ _ _ _ _ w102 _ _ _ _ _ _ _ _] -> w55
          tunnel: w52 -> [_ _ w76 _ _ _ _ w113 w133 w155 w175 w197 w212 w231]
          tunnel: w50 -> [w56 w67 w72 w84 w92 w99 w104 w109 w129 w152 w171 w198 w211 w230]
          tunnel: [w56 w67 w72 w81 w92 w100 w104 w108 w128 w151 w170 w190 w210 w229] -> w45
          tunnel: [_ _ _ _ _ _ _ w106 w126 w146 w168 w188 w207 w227] -> w44
          frame Default {
            # "'Default' case only runs if there is a message that isn't defined in any of the other cases.  Output a programming error."
            n167 = Format Into String(format string="The invalid message string \"%s\" was received in the Message Handling Loop." ("Invalid Message Loop Message"), w60) -> (resulting string=w57:string)  [unwired: 2 in, 1 out]
            n168 = call <vilib>:"Error Cluster From Error Code.vi"("error message (\"\")"=w57, "error code (0)"=1) -> ("error out"=w58:errorcluster)  [unwired: 7 in]
          }
          frame "Initialize" {
            n169 = call "Update Last State indicator value.vi"("error in (no error)"=w69, "Value"="Software Initialised") -> ("error out"=w65:errorcluster)  [unwired: 9 in]
            n170 = call "Enqueue Message.vi"("error in (no error)"=w65, "Message Data"="Ready" ("Ready..."), "Message"="Update Status", "Queue"=w66) -> ("error out"=w63:errorcluster)  [unwired: 6 in, 1 out]
            n171 = call "Ctrls state & value on Start-Stop.vi"("error in (no error)"=w63, "Queue data"=T13 {"Start/Stop"=enum."STOP", "State"=enum."Live Imaging-STOP"}) -> ("error out"=w62:errorcluster)  [unwired: 9 in]
          }
          frame "Update Status" {
            # "Update Display - Convert the message data to a string to display in the Status indicator."
            n172 = Variant To Data(error in=w77, type="", Variant=w76) -> (data=→"Status ind":string, error out=w73:errorcluster)
            n173 = Merge Errors(w73) -> (w78:errorcluster)
          }
          frame "Stop" {
            # "Stops the acquisition"
            # "Stop - Enable/Disable buttons appropriately for an acquisition that has stopped, and update status display."
            n174 = call "Enqueue Message.vi"("error in (no error)"=w83, "Message"="Stop", "Queue"=w84) -> ("error out"=w82:errorcluster, "Queue out"=w81:refnum<queue>)  [unwired: 7 in]
            n175 = call "Enqueue Message.vi"("error in (no error)"=w83, "Message Data"="Stopped" ("Ready..."), "Message"="Update Status", "Queue"=w88) -> ("error out"=w80:errorcluster)  [unwired: 6 in, 1 out]
            n176 = call <vilib>:"Clear Errors.vi"("error in (no error)"=w80) -> ("error out"=w79:errorcluster)  [unwired: 6 in]
            n177 = call "UI Cleanup.vi"("error in (no error)"=w79) -> ()  [unwired: 10 in, 1 out]
          }
          frame "Unload subpanel" {
            # "Update Display - Convert the message data to a string to display in the Status indicator."
            n178 = global read "General Globals.vi" "Subpanel is open"() -> (w91:bool)
            n179 = invoke on="Sub Panel" class="SubPnl" method="Remove VI"(error in=w90) -> (error out=w89:errorcluster)  [unwired: 2 in, 2 out]
            n180 = case shown="True" w91 {
              tunnel: w89 -> [w94 w96]
              tunnel: [w94 w96] -> w93
              frame False {
              }
              frame True {
                # "A subpanel is open"
                n181 = global write "General Globals.vi" "Stop subpanel"(TRUE ("Stop subpanel")) -> ()
              }
            }
          }
          frame "Exit" {
            w102 = TRUE
            # "Exit - Fire the User Event to stop the Event Handling Loop.  Also send Exit messages to the Acqusition and Logging loops."
            n182 = call "Exit case.vi"("error in"=w103, "UI queue"=w97, "Acq. queue"=w99) -> ("error out"=w101:errorcluster, "Exit String"=w98:string, "Acq. queue (out)"=w100:refnum<queue>)  [unwired: 6 in]
            n183 = local write "Status ind"(w98) -> ()
            "Stop" <- w102
          }
          frame "<IMAGING CASES BELOW>" {
          }
          frame "AOL Z Stack" {
            n184 = call "Variant to Data-Imaging protocol queue.vi"("error in (no error)"=w115, "Message Data"=w113) -> ("error out"=w114:errorcluster, "Next state queue data"=w106:T13)  [unwired: 8 in]
            n185 = Unbundle By Name(w106) -> ("Start/Stop"=w112:T14)
            n186 = case shown="\"STOP\", Default" w112 {
              tunnel: w116 -> [w117 _]
              tunnel: w114 -> [w118 w125]
              tunnel: w109 -> [w122 w124]
              tunnel: [w120 w125] -> w110
              tunnel: [w121 w124] -> w108
              tunnel: w107 -> [w119 _]
              frame "START" {
                n187 = call "Start Logic.vi"("error in (no error)"=w118, "Case name string"=w119, "UI queue"=w117, "Acq. queue in"=w122) -> ("error out"=w120:errorcluster, "Acq. queue"=w121:refnum<queue>)  [unwired: 6 in]
              }
              frame "STOP", Default {
                # "Place here (as a sub-VI) any code that you need to execute when the \"AOL Z Stack\" completes.\nUse the \"Fire User Event - Next State.vi\" to fire a programatic event and cause this case to execute."
                n188 = call "Pockels-manage mod setting.vi"("Function"=enum16{"Capture setting", "Re-apply setting"}."Re-apply setting") -> ()  [unwired: 10 in, 1 out]
              }
            }
            n189 = call "Ctrls state & value on Start-Stop.vi"("error in (no error)"=w110, "Queue data"=w106) -> ("error out"=w111:errorcluster)  [unwired: 9 in]
          }
          frame "Motor Z Stack" {
            n190 = call "Variant to Data-Imaging protocol queue.vi"("error in (no error)"=w135, "Message Data"=w133) -> ("error out"=w134:errorcluster, "Next state queue data"=w126:T13)  [unwired: 8 in]
            n191 = Unbundle By Name(w126) -> ("Start/Stop"=w132:T14)
            n192 = case shown="\"START\"" w132 {
              tunnel: [w139 w141] -> w130
              tunnel: w129 -> [w138 w145]
              tunnel: w136 -> [_ w143]
              tunnel: w134 -> [w139 w140]
              tunnel: [w138 w144] -> w128
              tunnel: w127 -> [_ w142]
              frame "STOP", Default {
                # "Place here (as a sub-VI) any code that you need to execute when the \"Motor Z Stack\" completes.\nUse the \"Fire User Event - Next State.vi\" to fire a programatic event and cause this case to execute."
                n193 = call "Pockels-manage mod setting.vi"("Function"=enum16{"Capture setting", "Re-apply setting"}."Re-apply setting") -> ()  [unwired: 10 in, 1 out]
              }
              frame "START" {
                n194 = call "Start Logic.vi"("error in (no error)"=w140, "Case name string"=w142, "UI queue"=w143, "Acq. queue in"=w145) -> ("error out"=w141:errorcluster, "Acq. queue"=w144:refnum<queue>)  [unwired: 6 in]
              }
            }
            n195 = call "Ctrls state & value on Start-Stop.vi"("error in (no error)"=w130, "Queue data"=w126) -> ("error out"=w131:errorcluster)  [unwired: 9 in]
          }
          frame "Live Imaging" {
            n196 = call "Variant to Data-Imaging protocol queue.vi"("error in (no error)"=w156, "Message Data"=w155) -> ("error out"=w148:errorcluster, "Next state queue data"=w146:T13)  [unwired: 8 in]
            n197 = call "Ctrls state & value on Start-Stop.vi"("error in (no error)"=w148, "Queue data"=w146) -> ("error out"=w147:errorcluster)  [unwired: 9 in]
            n198 = Unbundle By Name(w146) -> ("Start/Stop"=w154:T14)
            n199 = case shown="\"STOP\", Default" w154 {
              tunnel: w152 -> [w160 w163]
              tunnel: [w157 w166] -> w150
              tunnel: w149 -> [w159 w162]
              tunnel: w147 -> [w158 w165]
              tunnel: w153 -> [_ w161]
              tunnel: [w160 w164] -> w151
              frame "STOP", Default {
                n200 = call "Stop Logic-Imaging.vi"("error in (no error)"=w158, "UI queue"=w159) -> ("error out"=w157:errorcluster)  [unwired: 9 in]
              }
              frame "START" {
                n201 = call "Start Logic.vi"("error in (no error)"=w165, "Case name string"=w161, "UI queue"=w162, "Acq. queue in"=w163) -> ("error out"=w166:errorcluster, "Acq. queue"=w164:refnum<queue>)  [unwired: 6 in]
              }
            }
          }
          frame "Live volume imaging" {
            n202 = call "Variant to Data-Imaging protocol queue.vi"("error in (no error)"=w176, "Message Data"=w175) -> ("error out"=w167:errorcluster, "Next state queue data"=w168:T13)  [unwired: 8 in]
            n203 = Unbundle By Name(w168) -> ("Start/Stop"=w174:T14)
            n204 = case shown="\"START\"" w174 {
              tunnel: w177 -> [w178 w185]
              tunnel: w171 -> [w181 w187]
              tunnel: [w179 w182] -> w172
              tunnel: w167 -> [w180 w184]
              tunnel: [w181 w186] -> w170
              tunnel: w169 -> [_ w183]
              frame "STOP", Default {
                n205 = call "Stop Logic-Imaging.vi"("error in (no error)"=w180, "UI queue"=w178) -> ("error out"=w179:errorcluster)  [unwired: 9 in]
              }
              frame "START" {
                n206 = call "Start Logic.vi"("error in (no error)"=w184, "Case name string"=w183, "UI queue"=w185, "Acq. queue in"=w187) -> ("error out"=w182:errorcluster, "Acq. queue"=w186:refnum<queue>)  [unwired: 6 in]
              }
            }
            n207 = call "Ctrls state & value on Start-Stop.vi"("error in (no error)"=w172, "Queue data"=w168) -> ("error out"=w173:errorcluster)  [unwired: 9 in]
          }
          frame "Functional Acquisition" {
            n208 = call "Variant to Data-Imaging protocol queue.vi"("error in (no error)"=w196, "Message Data"=w197) -> ("error out"=w195:errorcluster, "Next state queue data"=w188:T13)  [unwired: 8 in]
            n209 = Unbundle By Name(w188) -> ("Start/Stop"=w193:T14)
            n210 = case shown="\"START\"" w193 {
              tunnel: w198 -> [w204 w205]
              tunnel: [w200 w206] -> w191
              tunnel: w195 -> [w199 w206]
              tunnel: w194 -> [w202 _]
              tunnel: [w203 w205] -> w190
              tunnel: w189 -> [w201 _]
              frame "START" {
                n211 = call "Start Logic.vi"("error in (no error)"=w199, "Case name string"=w201, "UI queue"=w202, "Acq. queue in"=w204) -> ("error out"=w200:errorcluster, "Acq. queue"=w203:refnum<queue>)  [unwired: 6 in]
              }
              frame "STOP", Default {
                n212 = call "Funct Acq Stop Actions.vi"() -> ()  [unwired: 12 in]
              }
            }
            n213 = call "Ctrls state & value on Start-Stop.vi"("error in (no error)"=w191, "Queue data"=w188) -> ("error out"=w192:errorcluster)  [unwired: 9 in]
          }
          frame "Single Plane Acquisition" {
            n214 = call "Variant to Data-Imaging protocol queue.vi"("error in (no error)"=w216, "Message Data"=w212) -> ("error out"=w215:errorcluster, "Next state queue data"=w207:T13)  [unwired: 8 in]
            n215 = Unbundle By Name(w207) -> ("Start/Stop"=w213:T14)
            n216 = case shown="\"START\"" w213 {
              tunnel: w217 -> [w221 _]
              tunnel: w211 -> [w223 w225]
              tunnel: w215 -> [w219 w226]
              tunnel: [w222 w225] -> w210
              tunnel: w209 -> [w220 _]
              tunnel: [w218 w226] -> w208
              frame "START" {
                n217 = call "Start Logic.vi"("error in (no error)"=w219, "Case name string"=w220, "UI queue"=w221, "Acq. queue in"=w223) -> ("error out"=w218:errorcluster, "Acq. queue"=w222:refnum<queue>)  [unwired: 6 in]
              }
              frame "STOP", Default {
                # "Place here (as a sub-VI) any code that you need to execute when the \"Single Plane Acquitition\" completes.\nUse the \"Fire User Event - Next State.vi\" to fire a programatic event and cause this case to execute."
                n218 = call "Pockels-manage mod setting.vi"("Function"=enum16{"Capture setting", "Re-apply setting"}."Re-apply setting") -> ()  [unwired: 10 in, 1 out]
              }
            }
            n219 = call "Ctrls state & value on Start-Stop.vi"("error in (no error)"=w208, "Queue data"=w207) -> ("error out"=w214:errorcluster)  [unwired: 9 in]
          }
          frame "Volume acquisition" {
            n220 = call "Variant to Data-Imaging protocol queue.vi"("error in (no error)"=w235, "Message Data"=w231) -> ("error out"=w234:errorcluster, "Next state queue data"=w227:T13)  [unwired: 8 in]
            n221 = Unbundle By Name(w227) -> ("Start/Stop"=w232:T14)
            n222 = case shown="\"STOP\", Default" w232 {
              tunnel: w230 -> [w242 w245]
              tunnel: [w240 w246] -> w236
              tunnel: w234 -> [w243 w246]
              tunnel: w233 -> [w239 _]
              tunnel: [w241 w245] -> w229
              tunnel: w228 -> [w238 _]
              frame "START" {
                n223 = call "Start Logic.vi"("error in (no error)"=w243, "Case name string"=w238, "UI queue"=w239, "Acq. queue in"=w242) -> ("error out"=w240:errorcluster, "Acq. queue"=w241:refnum<queue>)  [unwired: 6 in]
              }
              frame "STOP", Default {
                # "Place here (as a sub-VI) any code that you need to execute when the \"Volume acquisition\" completes.\nUse the \"Fire User Event - Next State.vi\" to fire a programatic event and cause this case to execute."
                n224 = call "Pockels-manage mod setting.vi"("Function"=enum16{"Capture setting", "Re-apply setting"}."Re-apply setting") -> ()  [unwired: 10 in, 1 out]
              }
            }
            n225 = call "Ctrls state & value on Start-Stop.vi"("error in (no error)"=w236, "Queue data"=w227) -> ("error out"=w237:errorcluster)  [unwired: 9 in]
          }
        }
        n226 = call "Error handler-UI handling loop.vi"("error in (no error)"=w49) -> ("No error"=w47:errorcluster)  [unwired: 10 in]
        n227 = call "Set status to Idle.vi"("Next state queue data"=w44, "UI queue"=w43) -> ()  [unwired: 10 in]
      }
      n228 = Unregister For Events(event registration refnum=w36) -> (error out=w25:errorcluster)  [unwired: 1 in]
      n229 = call <vilib>:"Clear Errors.vi"("error in (no error)"=w25) -> ()  [unwired: 6 in, 1 out]
      n230 = call "Compute Chirp Parameters.vi"("Error in"=w20) -> ("error out"=w29:errorcluster)  [unwired: 9 in, 1 out]
      n231 = call "Utility processes.vi"("error in (no error)"=w20) -> ("error out"=w19:errorcluster)  [unwired: 10 in]
      n232 = call "Acquisition Module.vi"("Error In"=w20, "Queues Cluster"=w38) -> ("Error Out"=w28:errorcluster)  [unwired: 9 in]
      n233 = call "Logging Module.vi"("Logging process enabled"=TRUE, "Data Queue error in"=w20, "Queues Cluster"=w38) -> ("error out"=w32:errorcluster)  [unwired: 8 in]
      n234 = call "Encoder Driver.vi"("UI elements cluster"=w18) -> ("Error out (no error)"=w31:errorcluster)  [unwired: 10 in]
      n235 = call "XYZ Stage Driver.vi"("UI elements cluster"=w18) -> ("error out (no error)"=w24:errorcluster)  [unwired: 10 in]
      n236 = Merge Errors(w26, w22, w29, w19, w28, w32, w31, w24) -> (w30:errorcluster)
      n237 = call "Software Cleanup.vi"("error in (no error)"=w30) -> ("error out"=w27:errorcluster)  [unwired: 10 in]
      n238 = flat-sequence {
        tunnel: w27 -> [_]
        frame #0 {
          n239 = Request Deallocation(TRUE ("flag")) -> ()
        }
        frame #1 {
          n240 = call "Close panel if exe-Top level VI.vi"() -> ()  [unwired: 11 in, 1 out]
        }
      }
    }
    frame True {
      # "Application shutting down due to lack of admin proviledges"
      n241 = global write "gl_UI Ctrl Refs.vi" "UI ctrl refs"(w319) -> ()
      n242 = flat-sequence {
        tunnel: w319 -> [_]
        frame #0 {
          n243 = call "Close panel if exe-Top level VI.vi"() -> ()  [unwired: 11 in, 1 out]
        }
      }
    }
  }
